vi "Query Multi Eval Meas List Segment DMRS Type B.vi"(0 "VISA resource name":refnum<visa-resource-name>, 1 "BWP (0)":i32, 5 "Instance (1)":T2=1, 7 "Segment (1)":i32=1, 9 "CC (1)":T1=1, 11 "error in (no error)":errorcluster) -> (4 "VISA resource name out":refnum<visa-resource-name>, 6 "Config Type":i32, 8 "Additional Position":i32, 10 "Max Length":i32, 15 "error out":errorcluster)   [LabVIEW 2020, in "Rohde&Schwarz CMWXP NR FR1 Measurement.lvlib"]
doc: "Queries the DM-RS for mapping type B. The settings apply to the <BWP> on carrier <cc> in segment <no>.\n\nAttribute:\n-\n\nRemote-control command:\nCONFigure:NRSub:MEAS<i>:LIST:SEGMent<no>[:CC<cc>]:BWPart:PUSCh:DMTB?"
uses:
  <instrlib>/Rohde&Schwarz CMWXP NR FR1 Measurement/Rohde&Schwarz CMWXP NR FR1 Measurement.lvlib
  <instrlib>/Rohde&Schwarz CMWXP NR FR1 Measurement/Private/_Instance.ctl
  <instrlib>/Rohde&Schwarz CMWXP NR FR1 Measurement/Private/_Carrier Component.ctl
  <instrlib>/Rohde&Schwarz CMWXP NR FR1 Measurement/Private/rsidr_core.llb/rsidr_core.lvlib
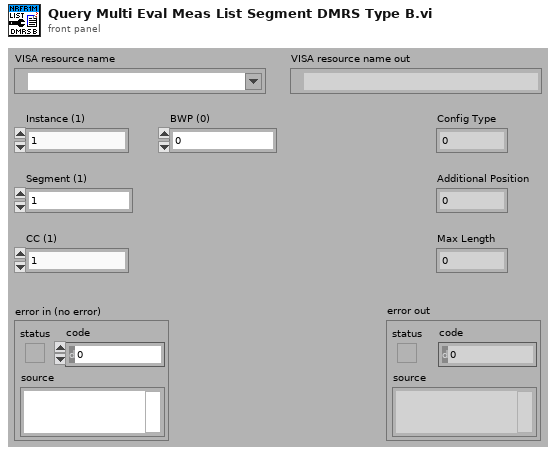
[diagram p1: front panel]
types:
  T1 = typedef "Rohde&Schwarz CMWXP NR FR1 Measurement.lvlib/_Carrier Component.ctl" = i32
  T2 = typedef "Rohde&Schwarz CMWXP NR FR1 Measurement.lvlib/_Instance.ctl" = i32
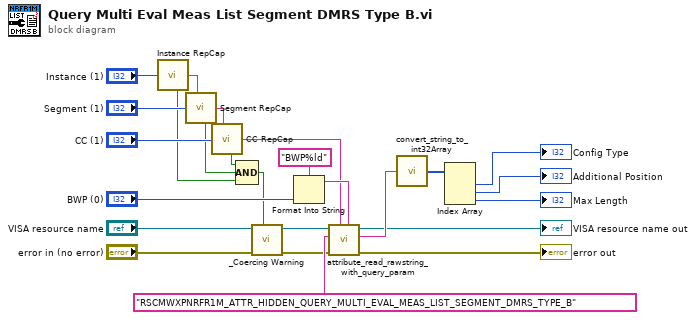
[diagram p0: block diagram]
diagram:
  n1 = call <instrlib>:"Instance RepCap.vi"("Instance In"="Instance (1)") -> ("In Range?"=w8:bool, "RepCap Identifier Out"=w21:string)  [unwired: 1 in]
  n2 = call <instrlib>:"Segment RepCap.vi"("Segment In"="Segment (1)", "RepCap String In (\"\")"=w21) -> ("In Range?"=w7:bool, "RepCap Identifier Out"=w22:string)
  n3 = call <instrlib>:"CC RepCap.vi"("CC In"="CC (1)", "RepCap String In (\"\")"=w22) -> ("In Range?"=w6:bool, "RepCap Identifier Out"=w17:string)
  n4 = Compound Arithmetic op=AND(w6, w7, w8) -> (w1:bool)
  n5 = call <instrlib>:"_Coercing Warning.vi"("In Range?"=w1, "error in (no error)"="error in (no error)", "VISA resource name"="VISA resource name") -> ("error out"=w3:errorcluster, "VISA resource name out"=w2:refnum<visa-resource-name>)  [unwired: 7 in]
  n6 = Format Into String(format string="BWP%ld", "BWP (0)") -> (resulting string=w18:string)  [unwired: 2 in, 1 out]
  n7 = call <instrlib>:"attribute_read_rawstring_with_query_param.vi"("Query Parameter (None)"=w18, "Repeated Capability"=w17, "error in"=w3, "Attribute ID"="RSCMWXPNRFR1M_ATTR_HIDDEN_QUERY_MULTI_EVAL_MEAS_LIST_SEGMENT_DMRS_TYPE_B", "VISA resource name"=w2) -> ("error out"=→"error out":errorcluster, "Raw String out"=w16:string, "VISA resource name out"=→"VISA resource name out":refnum<visa-resource-name>)  [unwired: 4 in]
  n8 = call <instrlib>:"convert_string_to_int32Array.vi"("string in"=w16) -> ("int32 array out"=w15:i32[])  [unwired: 3 in, 1 out]
  n9 = Index Array(array=w15) -> (element #1=→"Config Type":i32, element #2=→"Additional Position":i32, element #3=→"Max Length":i32)  [unwired: 3 in]
